vi "Extract Data 3.1.vi"(6 "Single/Permutations":bool, 7 "Settings":string, 8 "Error In":errorcluster, 9 "Search Path":path, 10 "File Search Phrase":string="Smoothness", 11 "Summary File Title":string="Subject Means") -> (0 "error out":errorcluster, 3 "Saved Path":string)   [LabVIEW 2020]
uses:
  <userlib>/_OpenG.lib/file/file.llb/File Exists - Scalar__ogtk.vi
  <vilib>/Analysis/NI_AALBase.lvlib
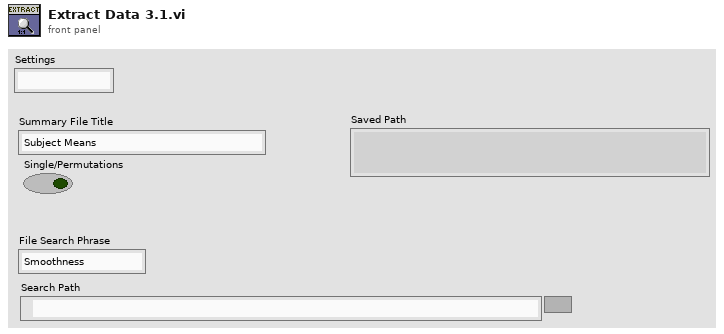
[diagram p1: front panel]
types:
  T1 = enum16{"open", "replace", "create", "open or create", "replace or create", "replace or create with confirmation"}
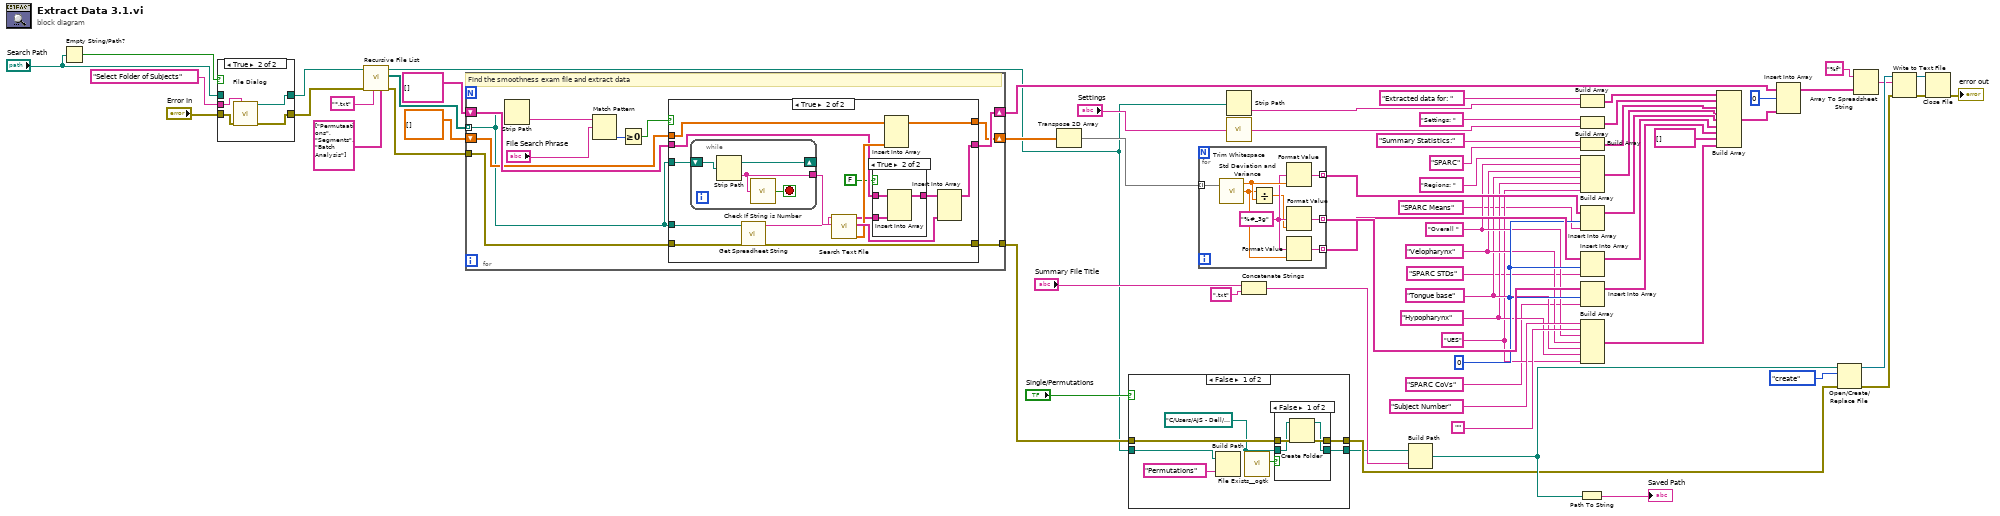
[diagram p0: block diagram]
diagram:
  w40 = 0 ("index")
  w19 = "UES" ("element")
  w20 = "Hypopharynx" ("element")
  w21 = "Tongue base" ("element")
  w22 = "Velopharynx" ("element")
  w23 = "Overall " ("element")
  n1 = Empty String/Path?(string/path="Search Path") -> (empty?=w29:bool)
  n2 = case shown="True" w29 {
    tunnel: "Error In" -> [w68 w73]
    tunnel: [w68 w72] -> w5
    tunnel: "Select Folder of Subjects" ("prompt") -> [_ w71]
    tunnel: [w69 w70] -> w7
    tunnel: "Search Path" -> [w69 _]
    frame False {
    }
    frame True {
      n3 = call "File Dialog"("prompt"=w71, "error in"=w73) -> ("selected path"=w70:path, "error out"=w72:errorcluster)  [unwired: 10 in, 2 out]
    }
  }
  n4 = call <vilib>:"Recursive File List.vi"("Folders to Exclude"=string[] ["Permutaations", "Segments", "Batch Analysis"], "pattern"="*.txt", "error in (no error)"=w5, "Folder Path"=w7) -> ("error out"=w2:errorcluster, "All Files in Dir"=w4:path[], "dup Folder Path"=w1:path)  [unwired: 3 in, 2 out]
  n5 = for {
    tunnel: w2 -> [w81]
    tunnel: [w80] -> w10
    shift-right: [w78] -> w49
    shift-left: string[][] [] ("appended array") -> [w79]
    tunnel: w4 -> [w74] mode=indexing
    shift-right: [w76] -> w52
    shift-left: dbl[][] [] -> [w77]
    # "Find the smoothness exam file and extract data"
    n6 = Strip Path(path=w74) -> (name=w75:string)  [unwired: 1 out]
    n7 = Match Pattern(string=w75, regular expression="File Search Phrase") -> (offset past match=w83:i32)  [unwired: 1 in, 3 out]
    n8 = Greater Or Equal To 0?(x=w83) -> (x >= 0?=w82:bool)
    n9 = case shown="True" w82 {
      tunnel: w81 -> [w87 w90]
      tunnel: [w87 w88] -> w80
      tunnel: w79 -> [w86 w97]
      tunnel: [w86 w102] -> w78
      tunnel: w77 -> [w85 w99]
      tunnel: [w85 w98] -> w76
      tunnel: w74 -> [_ w91]
      tunnel: w74 -> [_ w93]
      frame False {
      }
      frame True {
        n10 = while {
          shift-right: [w106] -> _
          shift-left: w93 -> [w105]
          tunnel: [w103] -> w92
          stop <- w104 stop-if-true
          n11 = Strip Path(path=w105) -> (stripped path=w106:path, name=w103:string)
          n12 = call "Check If String is Number.vi"("String"=w103) -> ("Is a Number?"=w104:bool)
        }
        n13 = call "Get Spreadheet String.vi"("error in (no error)"=w90, "File Path"=w91) -> ("error out"=w88:errorcluster, "Spreadsheet String"=w89:string)  [unwired: 8 in]
        n14 = call "Search Text File.vi"("Subject Number"=w92, "Spreadsheet String"=w89) -> ("SPARC Data"=w100:dbl[], "SPARC Data Text"=w101:string[], "NMD Data Text"=w96:string[])  [unwired: 6 in, 1 out]
        n15 = case shown="True" FALSE {
          tunnel: w97 -> [w107 w110]
          tunnel: w96 -> [_ w109]
          tunnel: [w107 w108] -> w95
          frame False {
          }
          frame True {
            n16 = Insert Into Array(array=w110, new element=w109) -> (w108:string[][])  [unwired: 2 in]
          }
        }
        n17 = Insert Into Array(array=w99, new element=w100) -> (w98:dbl[][])  [unwired: 2 in]
        n18 = Insert Into Array(array=w95, new element=w101) -> (w102:string[][])  [unwired: 2 in]
      }
    }
  }
  n19 = Transpose 2D Array(2D array=w52) -> (transposed array=w51:dbl[][])
  n20 = case shown="False" "Single/Permutations" {
    tunnel: w10 -> [w117 w124]
    tunnel: w1 -> [w116 w125]
    tunnel: [w113 w124] -> w9
    tunnel: [w112 w125] -> w8
    frame False {
      w111 = path "C:/Users/AJS - Dell/Desktop/Permutations" ("file path")
      n21 = Build Path(base path=w116, name or relative path="Permutations") -> ()  [unwired: 1 out]
      n22 = call-poly <userlib>:"File Exists__ogtk.vi"("file path"=w111) -> ("is directory"=w115:bool)  [unwired: 6 in, 1 out]
      n23 = case shown="False" w115 {
        tunnel: w117 -> [w121 w123]
        tunnel: [w120 w123] -> w113
        tunnel: w111 -> [w119 w122]
        tunnel: [w118 w122] -> w112
        frame False {
          n24 = Create Folder(path (use dialog)=w119, error in=w121) -> (created path=w118:path, error out=w120:errorcluster)  [unwired: 1 in, 1 out]
        }
        frame True {
        }
      }
    }
    frame True {
    }
  }
  n25 = for {
    tunnel: w51 -> [w133] mode=indexing
    tunnel: [w131] -> w43 mode=indexing
    tunnel: [w127] -> w42 mode=indexing
    tunnel: [w126] -> w41 mode=indexing
    w130 = "%#_3g" ("format string")
    n26 = call <vilib>:"Std Deviation and Variance.vi"("X"=w133) -> ("mean"=w132:dbl, "standard deviation"=w128:dbl)  [unwired: 1 in, 1 out]
    n27 = Divide(x=w128, y=w132) -> (x/y=w129:dbl)
    n28 = Format Value(format string=w130, value (0)=w132) -> (output string=w131:string)  [unwired: 1 in]
    n29 = Format Value(format string=w130, value (0)=w129) -> (output string=w127:string)  [unwired: 1 in]
    n30 = Format Value(format string=w130, value (0)=w128) -> (output string=w126:string)  [unwired: 1 in]
  }
  n31 = Strip Path(path=w1) -> (name=w54:string)  [unwired: 1 out]
  n32 = call <vilib>:"Trim Whitespace.vi"("string"="Settings") -> ("trimmed string"=w13:string)  [unwired: 1 in]
  n33 = Concatenate Strings("Summary File Title", ".txt" ("string")) -> (w60:string)
  n34 = Build Path(base path=w8, name or relative path=w60) -> (appended path=w31:path)
  n35 = Path To String(path=w31) -> (string=→"Saved Path":string)
  n36 = Build Array("Extracted data for: " ("input 1"), w54) -> (w27:string[])
  n37 = Build Array("Settings: " ("element"), w13) -> (w25:string[])
  n38 = Build Array("Summary Statistics:", "SPARC" ("element")) -> (w24:string[])
  n39 = Build Array("Regions: " ("element"), w23, w22, w21, w20, w19) -> (w18:string[])
  n40 = Insert Into Array(array=w43, index=w40, new element="SPARC Means" ("new element/subarray")) -> (w32:string[])
  n41 = Insert Into Array(array=w41, index=w40, new element="SPARC STDs" ("new element/subarray")) -> (w39:string[])
  n42 = Insert Into Array(array=w42, index=w40, new element="SPARC CoVs" ("new element/subarray")) -> (w38:string[])
  n43 = Build Array("Subject Number", "", w23, w22, w21, w20, w19) -> (w36:string[])
  n44 = Build Array(w27, w25, w24, w18, w32, w39, w38, string[] [] ("element"), w36) -> (w47:string[][])
  n45 = Insert Into Array(array=w49, index (row)=0, new element=w47) -> (w48:string[][])  [unwired: 1 in]
  n46 = Open/Create/Replace File(file path (use dialog)=w31, error in=w9, operation (0:open)=T1."create") -> (refnum out=w61:refnum<file>, error out=w57:errorcluster)  [unwired: 3 in, 1 out]
  n47 = Array To Spreadsheet String(array=w48, 3:"%f" ("format string")) -> (spreadsheet string=w56:string)  [unwired: 1 in]
  n48 = Write to Text File(file (use dialog)=w61, text=w56, error in=w57) -> (refnum out=w62:refnum<file>, error out=w63:errorcluster)  [unwired: 1 in, 1 out]
  n49 = Close File(refnum=w62, error in=w63) -> (error out=→"error out":errorcluster)  [unwired: 1 out]
